vi "4.vi"() -> ()   [LabVIEW 2015]
panel:
  out "Waveform Graph":dbl[](graph)=[29.229689631106226, 29.223112457917743, 29.22640104451137, 29.229689631106226, 29.22640104451137, 29.22640104451137, 29.22640104451137, 29.22640104451137, 29.232978217702314, 29.22640104451137, 29.22640104451137, 29.232978217702314, 29.229689631106226, 29.229689631106226, 29.22640104451137, 29.229689631106226, 29.22640104451137, 29.229689631106226, 29.223112457917743, 29.229689631106226, 29.229689631106226, 29.229689631106226, 29.229689631106226, 29.229689631106226, 29.229689631106226, 29.22640104451137, 29.21982387132535, 29.22640104451137, 29.22640104451137, 29.22640104451137, 29.22640104451137, 29.229689631106226, 29.229689631106226, 29.22640104451137, 29.223112457917743, 29.232978217702314, 29.229689631106226, 29.22640104451137, 29.229689631106226, 29.229689631106226, 29.223112457917743, 29.223112457917743, 29.22640104451137, 29.223112457917743, 29.22640104451137, 29.22640104451137, 29.232978217702314, 29.22640104451137, 29.223112457917743, 29.223112457917743, 29.229689631106226, 29.232978217702314, 29.22640104451137, 29.22640104451137, 29.229689631106226, 29.223112457917743, 29.22640104451137, 29.229689631106226, 29.22640104451137, 29.22640104451137, 29.223112457917743, 29.22640104451137, 29.22640104451137, 29.229689631106226, 29.22640104451137, 29.22640104451137, 29.229689631106226, 29.223112457917743, 29.22640104451137, 29.22640104451137, 29.223112457917743, 29.22640104451137, 29.22640104451137, 29.22640104451137, 29.22640104451137, 29.22640104451137, 29.22640104451137, 29.223112457917743, 29.22640104451137, 29.22640104451137, 29.229689631106226, 29.22640104451137, 29.223112457917743, 29.22640104451137, 29.229689631106226, 29.229689631106226, 29.22640104451137, 29.223112457917743, 29.232978217702314, 29.223112457917743, 29.223112457917743, 29.22640104451137, 29.229689631106226, 29.229689631106226, 29.223112457917743, 29.21982387132535, 29.22640104451137, 29.22640104451137, 29.223112457917743, 29.223112457917743]
  out "Waveform Chart":dbl(graph)=0.29223112457917744
  in  "physical channels":tag="Dev1/ai0"
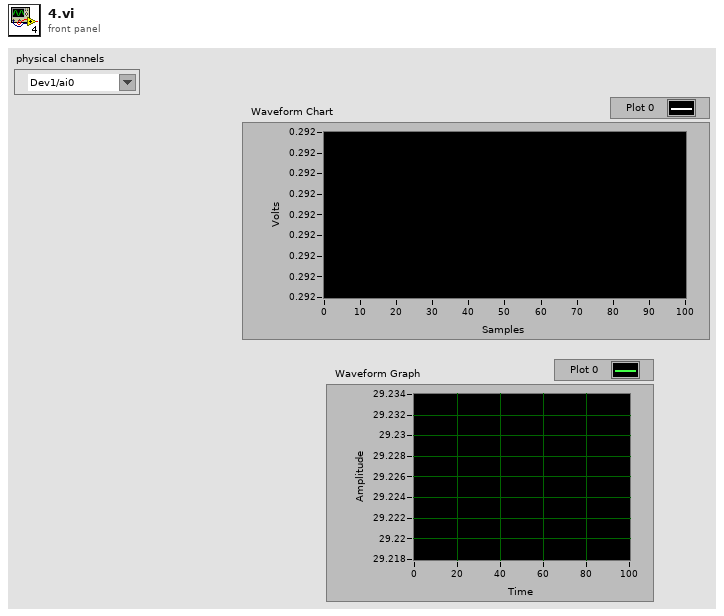
[diagram p1: front panel]
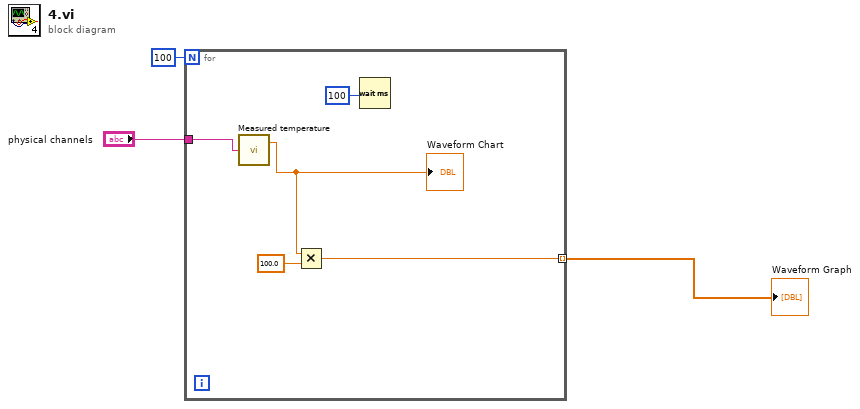
[diagram p0: block diagram]
diagram:
  n1 = for {
    N: 100 -> [_]
    tunnel: "physical channels" -> [w8]
    tunnel: [w4] -> w1 mode=indexing
    n2 = call "Measured temperature.vi"("physical channels"=w8) -> ("data"=w6:dbl)  [unwired: 1 out]
    "Waveform Chart" <- w6
    n3 = Multiply(x=w6, y=100.0) -> (x*y=w4:dbl)
    n4 = Wait (ms)(milliseconds to wait=u32 100) -> ()  [unwired: 1 out]
  }
  "Waveform Graph" <- w1
